vi "Scan Setup.vi"(8 "error in (no error)":errorcluster, 11 "multimeter reader in":refnum<class "multimeter reader.lvclass">) -> (0 "error out":errorcluster, 3 "multimeter reader out":refnum<class "multimeter reader.lvclass">)   [LabVIEW 2017, in "multimeter reader.lvclass"]
doc: "(Dynamic) Send commands to configure the instrument based on the class member fields."
uses:
  multimeter reader.lvclass
  Reader/Reader.lvclass
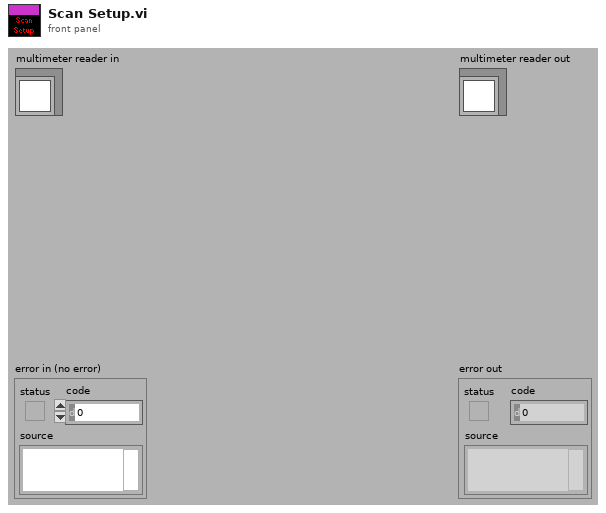
[diagram p1: front panel]
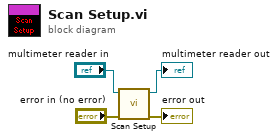
[diagram p0: block diagram]
diagram:
  n1 = call-parent "Scan Setup.vi"("error in (no error)"="error in (no error)", "Reader in"="multimeter reader in") -> ("error out"=→"error out":errorcluster, "Reader out"=→"multimeter reader out":refnum<class "multimeter reader.lvclass">)  [unwired: 8 in]
